vi "Execute Write Request.vi"(8 "error in (no error)":errorcluster, 10 "Write Request":refnum<class "WriteRequest.lvclass">, 11 "MultiplexedConnectionHandler in":refnum<class "MultiplexedConnectionHandler.lvclass">) -> (0 "error out":errorcluster, 3 "MultiplexedConnectionHandler out":refnum<class "MultiplexedConnectionHandler.lvclass">)   [LabVIEW 2019, in "MultiplexedConnectionHandler.lvlib" / "MultiplexedConnectionHandler.lvclass"]
uses:
  <vilib>/gpm_packages/@cs/Network-interface/Source/MultiplexedConnectionHandler/MultiplexedConnectionHandler/MultiplexedConnectionHandler.lvclass
  C:/Program Files/National Instruments/LabVIEW 2019/vi.lib/gpm_packages/@cs/Network-interface/Source/PersistantConnectionHandler/PersistantConnectionHandler/PersistantConnectionHandler.lvclass
  C:/Program Files/National Instruments/LabVIEW 2019/vi.lib/gpm_packages/@cs/Network-interface/Source/Logged Actor/LoggedActor.lvclass
  <vilib>/gpm_packages/@cs/Network-interface/Source/MessagingInterfaces/WriteRequest/WriteRequest.lvclass
  <vilib>/gpm_packages/@cs/Network-interface/Source/MultiplexedConnectionHandler/MultiplexedConnectionHandler/MultiplexedConnectionHandler.lvclass/MultiplexedConnectionHandler.ctl
  <vilib>/ActorFramework/Message Enqueuer/Message Enqueuer.lvclass
  <vilib>/gpm_packages/@cs/Network-interface/Source/Connection Reference/Connection Reference/Connection Reference.lvclass
  <vilib>/gpm_packages/@cs/event-logger/Source/Composed Log/Types/Log Level.ctl
  <vilib>/gpm_packages/@cs/Network-interface/Source/Logged Actor/LoggedActor.lvclass/LoggedActor.ctl
  <vilib>/gpm_packages/@cs/event-logger/Source/Composed Log/LoggerReference/LoggerReference.lvclass/LoggerReference.ctl
  <vilib>/gpm_packages/@cs/event-logger/Source/Composed Log/LoggerReference/Log Event.vi
  <vilib>/gpm_packages/@cs/event-logger/Source/Composed Log/LoggerReference/Log.vi
  <vilib>/gpm_packages/@cs/event-logger/Source/Composed Log/LoggerReference/Get Valid Event Time.vi
  <vilib>/gpm_packages/@cs/event-logger/Source/Composed Log/LoggerReference/Remove Stale Logs.vi
  <vilib>/ErrorRing/Error Ring.xnode
  <vilib>/gpm_packages/@cs/Network-interface/Source/PersistantConnectionHandler/PersistantConnectionHandler/PersistantConnectionHandler.lvclass
  <vilib>/gpm_packages/@cs/Network-interface/Source/Logged Actor/LoggedActor.lvclass
  <vilib>/gpm_packages/@cs/event-logger/Source/Composed Log/Composed Log.lvlib
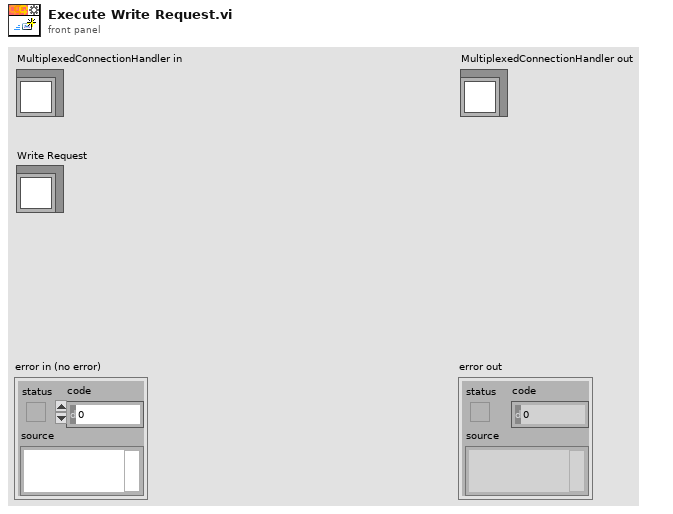
[diagram p1: front panel]
types:
  T1 = cluster{"Connection Manager Queue":refnum<class "Message Enqueuer.lvclass">, "Connection Reference":refnum<data-value>}
  T2 = typedef "Composed Log.lvlib/Log Level.ctl" = enum16{"Debug", "Info", "Warning", "Error", "Critical"}
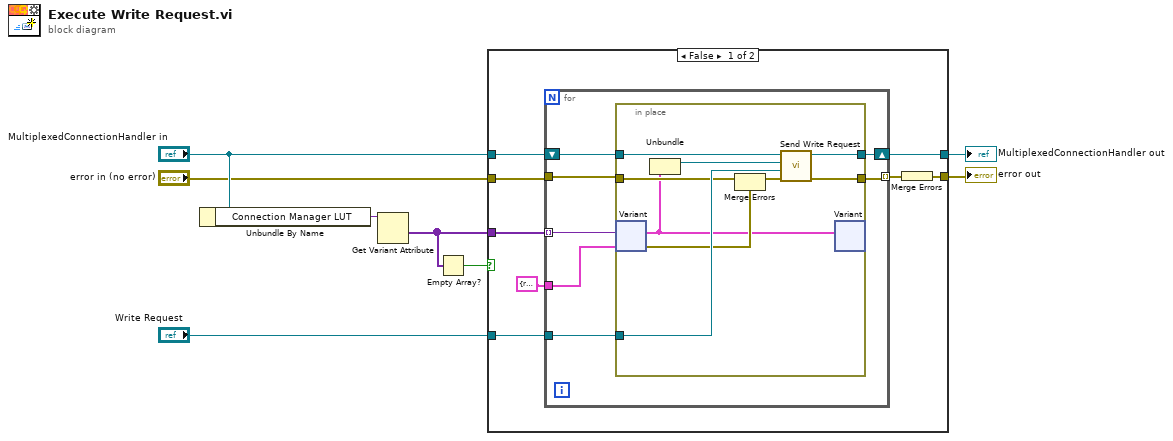
[diagram p0: block diagram]
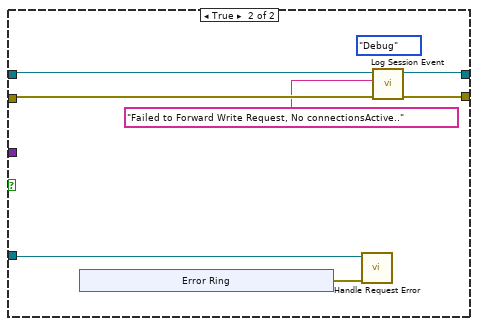
[diagram p2: hidden frame]
diagram:
  n1 = Unbundle By Name("MultiplexedConnectionHandler in") -> ("Connection Manager LUT"=w8:variant)
  n2 = Get Variant Attribute(Variant=w8) -> (values=w2:variant[])  [unwired: 3 in, 3 out]
  n3 = Empty Array?(array=w2) -> (empty?=w1:bool)
  n4 = case shown="False" w1 {
    tunnel: "MultiplexedConnectionHandler in" -> [w16 w39]
    tunnel: [w15 w37] -> w6
    tunnel: "Write Request" -> [w14 w34]
    tunnel: "error in (no error)" -> [w13 w38]
    tunnel: [w9 w36] -> w3
    tunnel: w2 -> [w10 _]
    frame False {
      n5 = for {
        tunnel: w10 -> [w21] mode=indexing
        shift-right: [w22] -> w15
        shift-left: w16 -> [w23]
        tunnel: T1 {"Connection Manager Queue"=refnum, "Connection Reference"=refnum} -> [w20]
        tunnel: w14 -> [w19]
        tunnel: w13 -> [w18]
        tunnel: [w17] -> w12 mode=indexing
        n6 = in-place {
          in-place-border: w23 -> [w32]
          in-place-border: [w31] -> w22
          in-place-border: w19 -> [w30]
          in-place-border: w18 -> [w29]
          in-place-border: [w28] -> w17
          n7 = in-place-variant #1(w21, w20) -> (w25:T1, w26:errorcluster)
          n8 = Unbundle(w25) -> ("Connection Manager Queue"=w24:refnum<class "Message Enqueuer.lvclass">)  [unwired: 1 out]
          n9 = Merge Errors(w29, w26) -> (w27:errorcluster)
          n10 = call <vilib>:"Send Write Request.vi"("error in (no error)"=w27, "Write Request"=w30, "Connection Manager Queue"=w24, "PersistantConnectionHandler in"=w32) -> ("error out"=w28:errorcluster, "PersistantConnectionHandler out"=w31:refnum<class "MultiplexedConnectionHandler.lvclass">)  [unwired: 6 in]
          n11 = in-place-variant #1(w25) -> ()  [unwired: 2 out]
        }
      }
      n12 = Merge Errors(w12) -> (w9:errorcluster)
    }
    frame True {
      (unwired) Log_Level."Debug" ("Event Level")
      n13 = xnode "Error Ring"() -> ("error out"=w33:errorcluster)
      n14 = call-dynamic "Handle Request Error.vi"("Request Error"=w33, "WriteRequest in"=w34) -> ()  [unwired: 10 in]
      n15 = call <vilib>:"Log Session Event.vi"("error in (no error)"=w38, "Event Data"="Failed to Forward Write Request, No connectionsActive..", "SessionActor in"=w39) -> ("error out"=w36:errorcluster, "SessionActor out"=w37:refnum<class "MultiplexedConnectionHandler.lvclass">)  [unwired: 7 in]
    }
  }
  "error out" <- w3
  "MultiplexedConnectionHandler out" <- w6
